vi "RTD and PT index split.vi"(8 "error in (no error)":errorcluster, 11 "config":T1={"AO config"=[], "AI config"=[], "DI config"=[], "DO config"=[], "TC config"=[], "ACC config"=[], "SG config"=[], "Strain Gauge Settings"={"poisson ratio"=0.3, "nominal gage resistance"=120.0, "gage factor"=2.08}, "bridge information"={"strain configuration"=10271, "lead wire resistance"=1.7, "initial bridge voltage"=0.0, "voltage excitation source"=10200, "voltage excitation value"=3.3}, "Sample Rate"={"AI Sample Rate"=0.0, "AO Sample Rate"=0.0, "DI Sample Rate"=0.0, "TC Sample Rate"=0.0, "DO Sample Rate"=0.0, "SG Sample Rate"=0.0, "ACC Sample Rate"=0.0}} {"bridge information"."initial bridge voltage" format="%0.2f"; "bridge information"."voltage excitation source" items=["Internal"=10200, "External"=10167, "None"=10230]; "bridge information"."voltage excitation value" format="%0.2f"; "bridge information"."lead wire resistance" format="%0.2f"; "bridge information"."strain configuration" items=["Full Bridge I"=10183, "Full Bridge II"=10184, "Full Bridge III"=10185, "Half Bridge I"=10188, "Half Bridge II"=10189, "Quarter Bridge I"=10271, "Quarter Bridge II"=10272]; "ACC config"."Terminal configuration" items=["default"=-1, "RSE"=10083, "NRSE"=10078, "Differential"=10106, "Pseudodifferential"=12529]; "ACC config"."Sensitivity units" items=["mVolts/g"=12509, "Volts/g"=12510]; "TC config"."type" items=["J"=10072, "K"=10073, "N"=10077, "R"=10082, "S"=10085, "T"=10086, "B"=10047, "E"=10055]; "TC config"."units" items=["Deg C", "Deg F", "Kelvins", "Deg R", "From Custom Scale"]}) -> (0 "error out":errorcluster, 1 "RTD":i32[](array[numeric]))   [LabVIEW 2022 SP3]
uses:
  Controls/Config.ctl
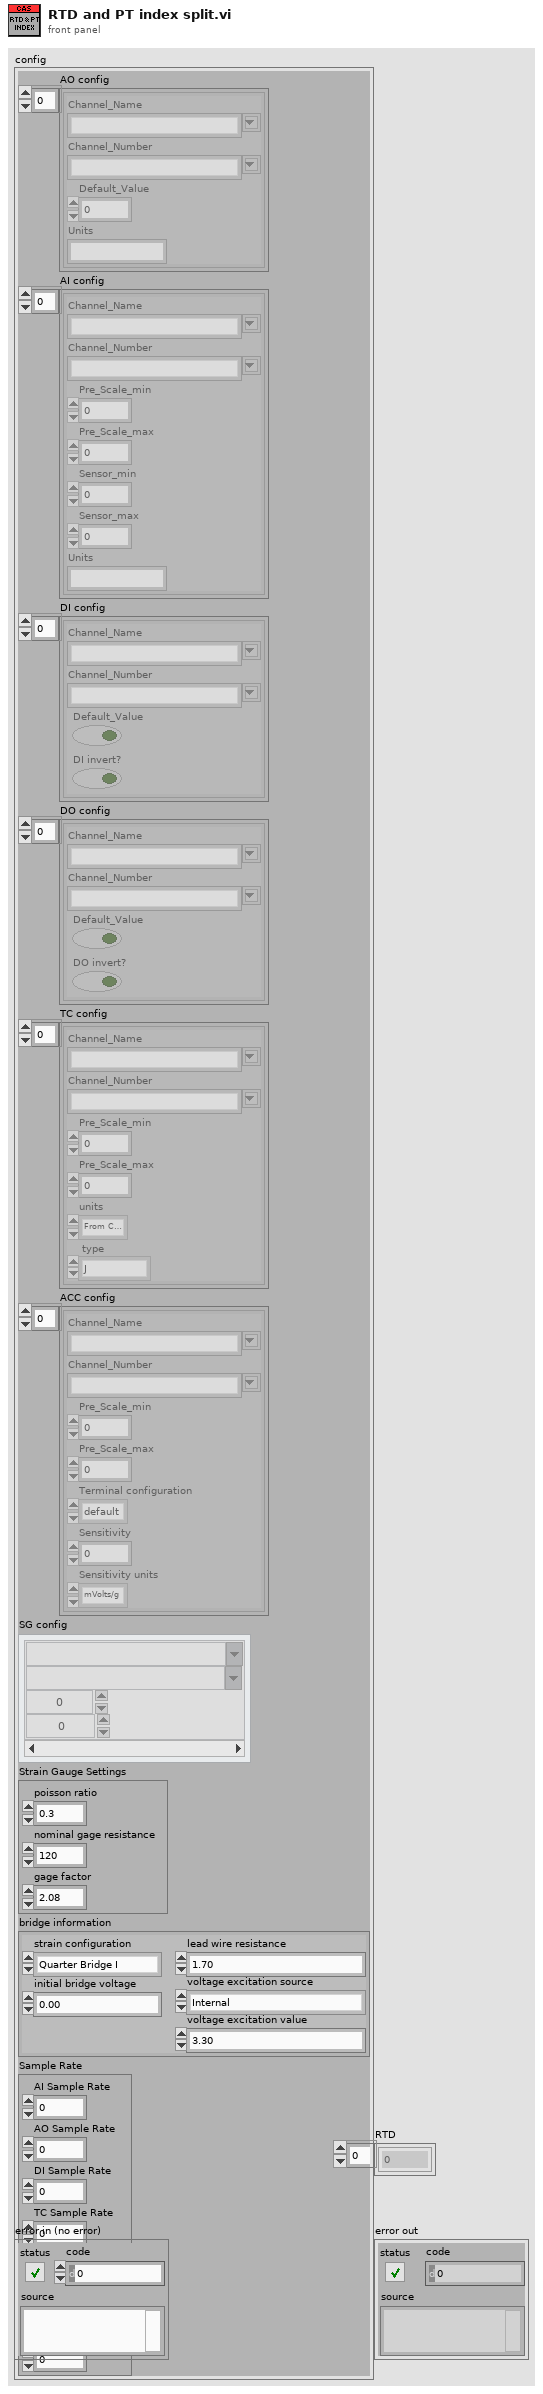
[diagram p1: front panel]
types:
  T1 = typedef "Config.ctl" = cluster{"AO config":cluster{"Channel_Name":string, "Channel_Number":string, "Default_Value":dbl, "Units":string}[], "AI config":cluster{"Channel_Name":string, "Channel_Number":string, "Pre_Scale_min":dbl, "Pre_Scale_max":dbl, "Sensor_min":dbl, "Sensor_max":dbl, "Units":string}[], "DI config":cluster{"Channel_Name":string, "Channel_Number":string, "Default_Value":bool, "DI invert?":bool}[], "DO config":cluster{"Channel_Name":string, "Channel_Number":string, "Default_Value":bool, "DO invert?":bool}[], "TC config":cluster{"Channel_Name":string, "Channel_Number":string, "Pre_Scale_min":dbl, "Pre_Scale_max":dbl, "units":i32, " type":i32}[], "ACC config":cluster{"Channel_Name":string, "Channel_Number":string, "Pre_Scale_min":dbl, "Pre_Scale_max":dbl, "Terminal configuration":i32, "Sensitivity":dbl, "Sensitivity units":i32}[], "SG config":cluster{"Channel_Name":string, "Channel_Number":string, "Pre_Scale_min":dbl, "Pre_Scale_max":dbl}[], "Strain Gauge Settings":cluster{"poisson ratio":dbl, "nominal gage resistance":dbl, "gage factor":dbl}, "bridge information":cluster{"strain configuration":i32, "lead wire resistance":dbl, "initial bridge voltage":dbl, "voltage excitation source":i32, "voltage excitation value":dbl}, "Sample Rate":cluster{"AI Sample Rate":dbl, "AO Sample Rate":dbl, "DI Sample Rate":dbl, "TC Sample Rate":dbl, "DO Sample Rate":dbl, "SG Sample Rate":dbl, "ACC Sample Rate":dbl}}
  T2 = cluster{"Channel_Name":string, "Channel_Number":string, "Pre_Scale_min":dbl, "Pre_Scale_max":dbl, "Sensor_min":dbl, "Sensor_max":dbl, "Units":string}[]
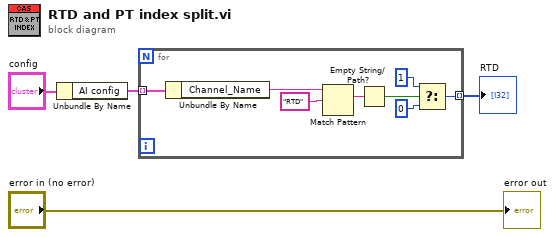
[diagram p0: block diagram]
diagram:
  n1 = Unbundle By Name("config") -> ("AI config"=w3:T2)
  n2 = for {
    tunnel: w3 -> [w12] mode=indexing
    tunnel: [w5] -> w1 mode=indexing
    n3 = Unbundle By Name(w12) -> ("Channel_Name"=w11:string)
    n4 = Match Pattern(string=w11, regular expression="RTD") -> (match substring=w9:string)  [unwired: 1 in, 3 out]
    n5 = Empty String/Path?(string/path=w9) -> (empty?=w8:bool)
    n6 = Select(t=1, s=w8, f=0) -> (s? t:f=w5:i32)
  }
  "RTD" <- w1
  "error out" <- "error in (no error)"
